vi "4431 USB - Create IO Channels.vi"(0 "sample mode":i32(ring)=10178 items=["Finite Samples"=10178, "Continuous Samples"=10123], 6 "error in":errorcluster, 7 "AI Buffer Size (S)":i32=10, 8 "sampling info":cluster{"Fs":dbl, "#s":dbl}, 9 "AO":T1={"AO amp (V)"=[0.1, 0.09, 0.08, 0.07, 0.06, 0.05, 0.04, 0.03], "AO DC (V)"=[0.0, 0.0, 0.0, 0.0, 0.0, 0.0, 0.0, 0.0], "AO f (Hz)"=[13.0, 13.0, 13.0, 13.0, 13.0, 13.0, 13.0, 13.0], "AO phi (deg)"=[0.0, 0.0, 0.0, 0.0, 0.0, 0.0, 0.0, 0.0], "function"=[enum."Sine Wave", enum."Sine Wave", enum."Sine Wave", enum."Sine Wave", enum."Sine Wave", enum."Sine Wave", enum."Sine Wave", enum."Sine Wave"]} {"AO DC (V)" format="%#_6p"; "AO amp (V)" format="%#_6p"}, 10 "AO Configuration":T2(array[cluster]), 11 "AI Configuration":T3(array[cluster])) -> (2 "AO Task":refnum<k21>[](array[refnum]), 3 "AI task":refnum<k21>[](array[refnum]), 4 "error out":errorcluster)   [LabVIEW 2016, in "SynchIO.USB4431.lvclass"]
uses:
  SynchIO.USB4431.lvclass
  <vilib>/DAQmx/read.llb/DAQmx Read (Analog 1D Wfm NChan NSamp).vi
  <vilib>/DAQmx/write.llb/DAQmx Write (Analog 1D Wfm NChan NSamp).vi
  <vilib>/DAQmx/create/channels.llb/DAQmx Create Channel (AO-Voltage-Basic).vi
  <vilib>/DAQmx/create/channels.llb/DAQmx Create Channel (AI-Voltage-Basic).vi
  <vilib>/DAQmx/configure/timing.llb/DAQmx Timing (Sample Clock).vi
  <vilib>/DAQmx/configure/trigger.llb/DAQmx Start Trigger (Digital Edge).vi
  <vilib>/DAQmx/miscellaneous.llb/DAQmx Fill In Error Info.vi
  <resource>/objmgr/daqmx.rc
panel:
  in  "AI.FilterDelay":dbl
  in  "AI.Gain":dbl
  in  "input terminal configuration":i32(ring)=-1 items=["default"=-1, "RSE"=10083, "NRSE"=10078, "Differential"=10106, "Pseudodifferential"=12529]
  in  "output terminal configuration":i32(ring)=-1 items=["Default"=-1, "RSE"=10083, "Differential"=10106, "Pseudodifferential"=12529]
  in  "SampClk.Timebase.Rate":dbl
  in  "SampQuant.SampPerChan":dbl
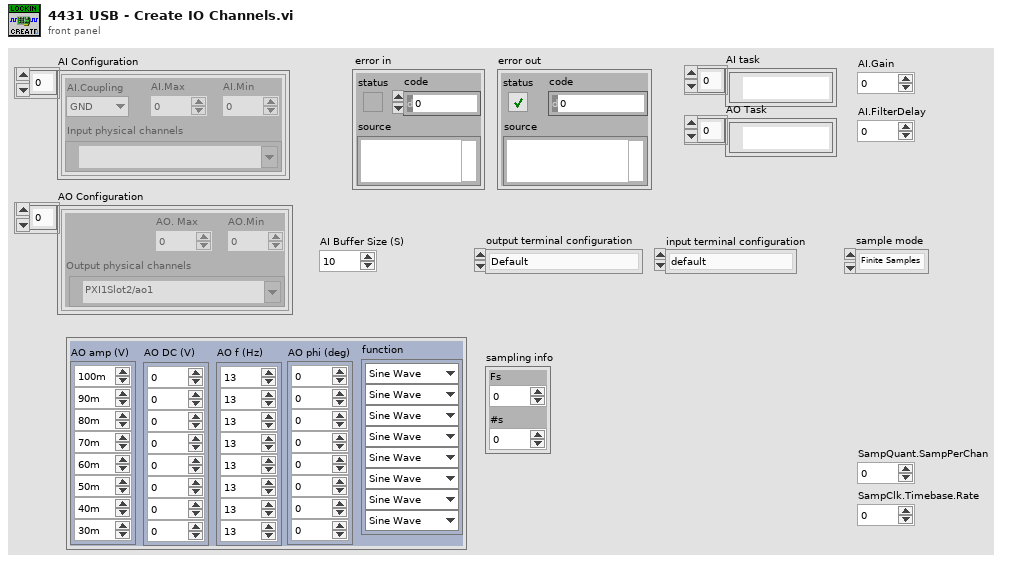
[diagram p1: front panel]
types:
  T1 = cluster{"AO amp (V)":dbl[], "AO DC (V)":dbl[], "AO f (Hz)":dbl[], "AO phi (deg)":dbl[], "function":enum16{"Sine Wave", "Triangle Wave", "Square Wave", "Sawtooth Wave"}[]}
  T2 = cluster{"Output physical channels":tag, "AO. Max":dbl, "AO.Min":dbl}[]
  T3 = cluster{"AI.Coupling":enum16{"AC", "DC", "GND"}, "AI.Max":dbl, "AI.Min":dbl, "Input physical channels":tag}[]
  T4 = cluster{"AI.Coupling":enum16{"AC", "DC", "GND"}, "AI.Max":dbl, "AI.Min":dbl, "Input physical channels":tag}
  T5 = cluster{"Output physical channels":tag, "AO. Max":dbl, "AO.Min":dbl}
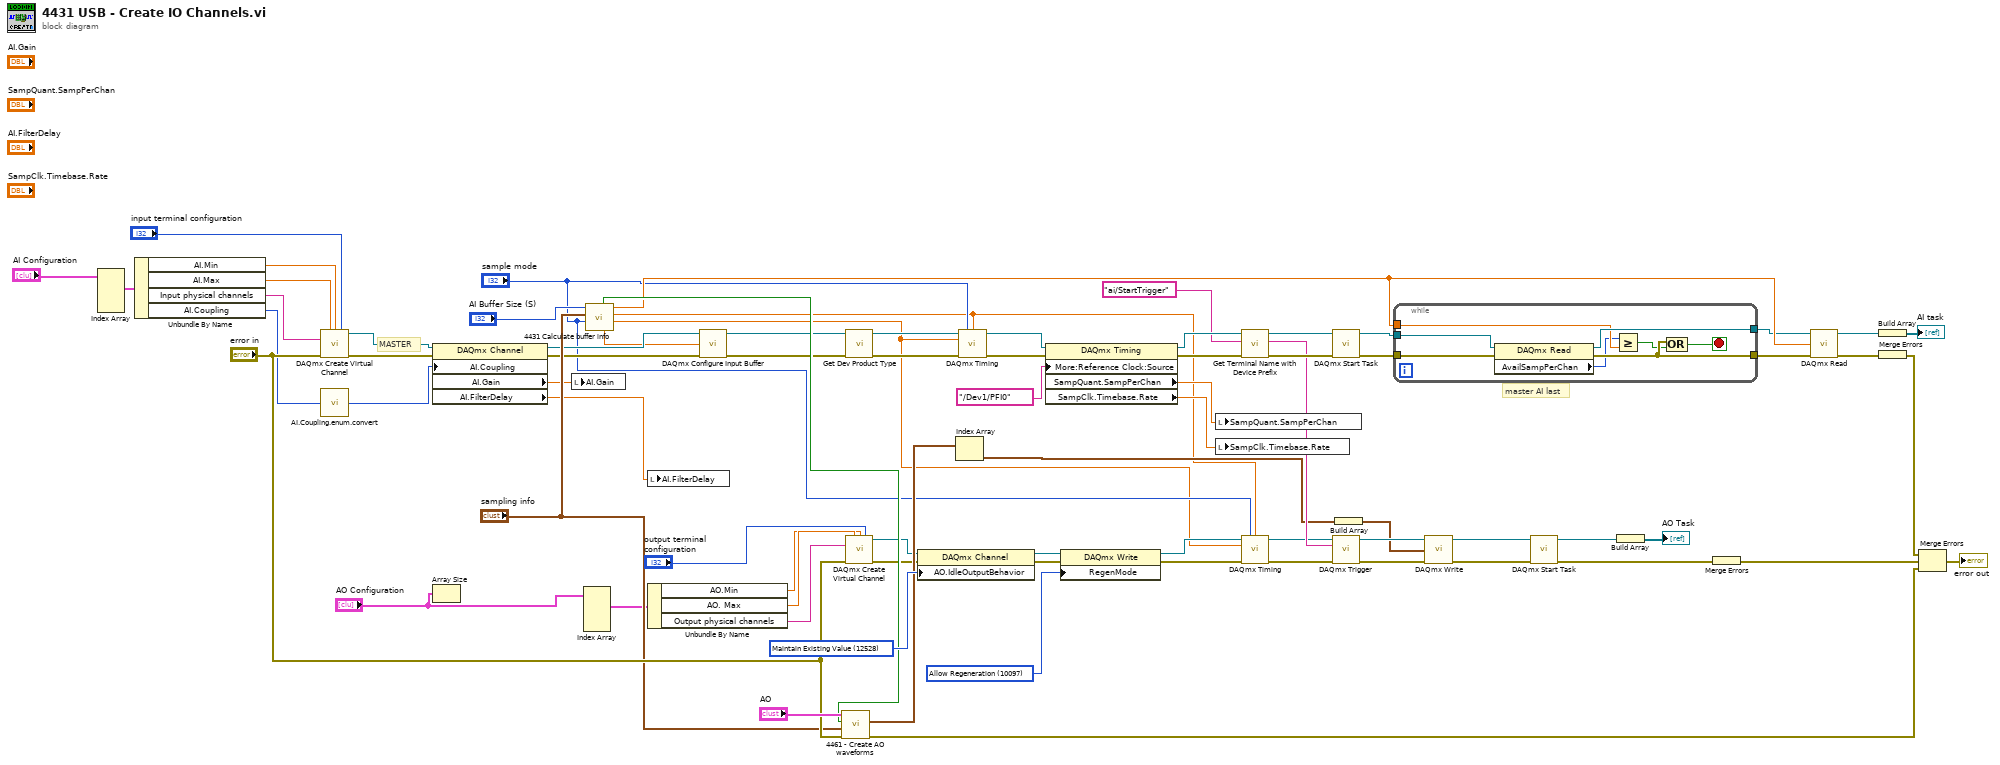
[diagram p0: block diagram]
diagram:
  w65 = 10097 items=["Allow Regeneration"=10097, "Do Not Allow Regeneration"=10158] ("RegenMode")
  w66 = 12528 items=["Zero Volts"=12526, "High-Impedance"=12527, "Maintain Existing Value"=12528] ("AO.IdleOutputBehavior")
  # "MASTER"
  # "master AI last"
  n1 = Index Array(array="AI Configuration") -> (element #1=w23:T4)  [unwired: 4 in, 3 out]
  n2 = Unbundle By Name(w23) -> ("AI.Min"=w18:dbl, "AI.Max"=w19:dbl, "Input physical channels"=w22:tag, "AI.Coupling"=w15:enum16{"AC", "DC", "GND"})
  n3 = call-poly <vilib>:"DAQmx Create Virtual Channel.vi"("maximum value"=w19, "minimum value"=w18, "input terminal configuration"="input terminal configuration", "physical channels"=w22, "error in"="error in") -> ("task out"=w21:refnum<k21>, "error out"=w20:errorcluster)  [unwired: 9 in]
  n4 = call "AI.Coupling.enum.convert.vi"("AI.Coupling"=w15) -> ("Numeric"=w14:i32)
  n5 = property class="DAQmx Channel"(reference=w21, error in=w20, "AI.Coupling"=w14) -> (reference out=w37:refnum<k21>, error out=w36:errorcluster, "AI.Gain"=w17:dbl, "AI.FilterDelay"=w16:dbl)
  n6 = Array Size(array="AO Configuration") -> ()  [unwired: 1 out]
  n7 = local write "AI.Gain"(w17) -> ()
  n8 = Index Array(array="AO Configuration") -> (element #1=w9:T5)  [unwired: 4 in, 3 out]
  n9 = call "4431 Calculate buffer info.vi"("sample mode"="sample mode", "sampling info"="sampling info", "AI Buffer Size (S)"="AI Buffer Size (S)") -> ("Fs"=w26:dbl, "Numeric 2"=w25:dbl, "Numeric 3"=w62:dbl, "Numeric"=w24:dbl, "Boolean"=w64:bool)  [unwired: 4 in]
  n10 = local write "AI.FilterDelay"(w16) -> ()
  n11 = Unbundle By Name(w9) -> ("AO.Min"=w6:dbl, "AO. Max"=w7:dbl, "Output physical channels"=w8:tag)
  n12 = call <vilib>:"DAQmx Configure Input Buffer.vi"("task/channels in"=w37, "buffer size (in samples per channel)"=w24, "error in"=w36) -> ("task out"=w13:refnum<k21>, "error out"=w12:errorcluster)  [unwired: 11 in]
  n13 = call "4461 - Create AO waveforms.vi"("error in (no error)"="error in", "sampling info"="sampling info", "reset signal"=w64, "AO"="AO") -> ("error out"=w28:errorcluster, "AO Array"=w48:waveform(dbl)[])  [unwired: 4 in, 2 out]
  n14 = call "Get Dev Product Type.vi"("error in (no error)"=w12, "Refnum in"=w13) -> ("error out"=w33:errorcluster, "Refnum out"=w32:refnum<k21>)  [unwired: 7 in, 1 out]
  n15 = call-poly <vilib>:"DAQmx Create Virtual Channel.vi"("maximum value"=w7, "minimum value"=w6, "output terminal configuration"="output terminal configuration", "physical channels"=w8, "error in"="error in") -> ("task out"=w5:refnum<k21>, "error out"=w4:errorcluster)  [unwired: 9 in]
  n16 = property class="DAQmx Channel"(reference=w5, error in=w4, "AO.IdleOutputBehavior"=w66) -> (reference out=w3:refnum<k21>, error out=w2:errorcluster)
  n17 = Index Array(array=w48) -> (element=w49:waveform(dbl))  [unwired: 1 in]
  n18 = call-poly <vilib>:"DAQmx Timing.vi"("task/channels in"=w32, "sample mode"="sample mode", "samples per channel"=w25, "rate"=w26, "error in"=w33) -> ("task out"=w59:refnum<k21>, "error out"=w56:errorcluster)  [unwired: 9 in]
  n19 = property class="DAQmx Timing"(reference=w59, error in=w56, "More:Reference Clock:Source"=tag "/Dev1/PFI0" ("RefClk.Src")) -> (reference out=w51:refnum<k21>, error out=w31:errorcluster, "SampQuant.SampPerChan"=w39:dbl, "SampClk.Timebase.Rate"=w38:dbl)
  n20 = property class="DAQmx Write"(reference=w3, error in=w2, "RegenMode"=w65) -> (reference out=w47:refnum<k21>, error out=w45:errorcluster)
  n21 = local write "SampQuant.SampPerChan"(w39) -> ()
  n22 = local write "SampClk.Timebase.Rate"(w38) -> ()
  n23 = call "Get Terminal Name with Device Prefix.vi"("error in (no error)"=w31, "Local Terminal Name"="ai/StartTrigger", "task/channels in"=w51) -> ("error out"=w58:errorcluster, "Terminal Name with Device Prefix"=w55:tag, "task out"=w57:refnum<k21>)  [unwired: 6 in]
  n24 = call-poly <vilib>:"DAQmx Timing.vi"("task/channels in"=w47, "sample mode"="sample mode", "samples per channel"=w25, "rate"=w26, "error in"=w45) -> ("task out"=w46:refnum<k21>, "error out"=w30:errorcluster)  [unwired: 9 in]
  n25 = call <vilib>:"DAQmx Start Task.vi"("task/channels in"=w57, "error in"=w58) -> ("task out"=w43:refnum<k21>, "error out"=w35:errorcluster)  [unwired: 12 in]
  n26 = call-poly <vilib>:"DAQmx Trigger.vi"("task/channels in"=w46, "source"=w55, "error in"=w30) -> ("task out"=w54:refnum<k21>, "error out"=w53:errorcluster)  [unwired: 11 in]
  n27 = Build Array(w49) -> (w50:waveform(dbl)[])
  n28 = while {
    tunnel: w43 -> [w84]
    tunnel: w35 -> [w83]
    tunnel: [w79] -> w42
    tunnel: [w82] -> w44
    tunnel: w62 -> [w81]
    stop <- w80 stop-if-true
    n29 = property class="DAQmx Read"(reference=w84, error in=w83) -> (reference out=w82:refnum<k21>, error out=w79:errorcluster, "AvailSampPerChan"=w78:u32)
    n30 = Greater Or Equal?(x=w78, y=w81) -> (x >= y?=w77:bool)
    n31 = Compound Arithmetic op=OR(w79, w77) -> (w80:bool)
  }
  n32 = call-poly <vilib>:"DAQmx Write.vi"("task/channels in"=w54, "data"=w50, "error in"=w53) -> ("task out"=w61:refnum<k21>, "error out"=w60:errorcluster)  [unwired: 10 in, 1 out]
  n33 = call <vilib>:"DAQmx Start Task.vi"("task/channels in"=w61, "error in"=w60) -> ("task out"=w52:refnum<k21>, "error out"=w41:errorcluster)  [unwired: 12 in]
  n34 = Build Array(w52) -> (→"AO Task":refnum<k21>[])
  n35 = Merge Errors(w41) -> (w40:errorcluster)
  n36 = call-poly <vilib>:"DAQmx Read.vi"("task/channels in"=w44, "number of samples per channel"=w62, "error in"=w42) -> ("task out"=w11:refnum<k21>, "error out"=w10:errorcluster)  [unwired: 10 in, 1 out]
  n37 = Build Array(w11) -> (→"AI task":refnum<k21>[])
  n38 = Merge Errors(w10) -> (w29:errorcluster)
  n39 = Merge Errors(w29, w40, w28) -> (→"error out":errorcluster)
